vi "Progress_Bar_Start.vi"() -> ()   [LabVIEW 2016]
uses:
  <vilib>/Utility/miscctls.llb/LVBoundsTypeDef.ctl
panel:
  out "2D Picture":picture
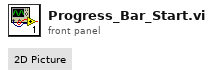
[diagram p1: front panel]
types:
  T1 = cluster{"left":i16, "top":i16, "right":i16, "bottom":i16}
  T2 = typedef "LVBoundsTypeDef.ctl" = cluster{"Width":u32, "Height":u32}
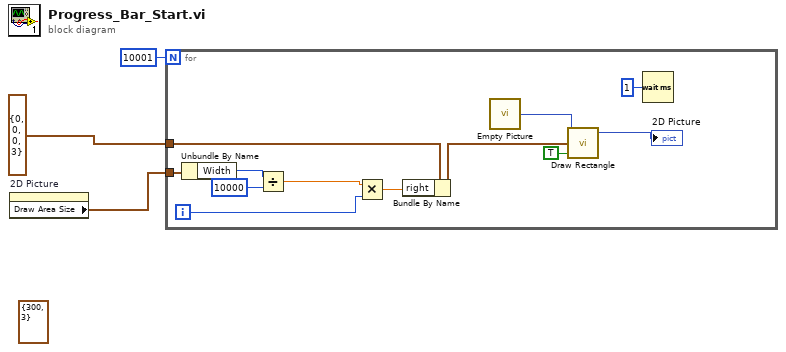
[diagram p0: block diagram]
diagram:
  (unwired) T2 {"Width"=300, "Height"=3} ("Draw Area Size")
  n1 = property on="2D Picture" class="Pict"() -> ("Draw Area Size"=w1:T2)  [unwired: 2 in, 2 out]
  n2 = for {
    N: 10001 -> [_]
    tunnel: T1 {"left"=0, "top"=0, "right"=0, "bottom"=3} ("rect") -> [w11]
    tunnel: w1 -> [w7]
    i -> [w12]
    n3 = Unbundle By Name(w7) -> ("Width"=w6:u32)
    n4 = Divide(x=w6, y=u32 10000) -> (x/y=w4:dbl)
    n5 = Multiply(x=w4, y=w12) -> (x*y=w9:dbl)
    n6 = Bundle By Name(cluster=w11, "right"=w9) -> (w10:T1)
    n7 = call "Empty Picture"() -> ("empty picture"=w14:picture)
    n8 = call <vilib>:"Draw Rectangle.vi"("picture"=w14, "rect"=w10, "fill?(F)"=TRUE) -> ("new picture"=→"2D Picture":picture)  [unwired: 6 in]
    n9 = Wait (ms)(milliseconds to wait=u32 1) -> ()  [unwired: 1 out]
  }
